vi "Get Attributes.vi"(0 "Linked List in":refnum<class "Linked List.lvclass">, 1 "Unique ID":string, 2 "Include Private?":bool, 3 "Flatten Pointer?":bool, 5 "Attribute Names":string[](array[string]), 7 "Missing GUIDs":string[](array[string]), 9 "Type":variant, 11 "error in (no error)":errorcluster) -> (4 "Linked List out":refnum<class "Linked List.lvclass">, 6 "Attribute Names out":string[](array[string]), 8 "Missing GUIDs out":string[](array[string]), 10 "Attributes":variant[](array[variant]), 12 "Found?":bool[](array[boolean]), 14 "Data IDs":string[](array[string]), 15 "error out":errorcluster)   [LabVIEW 2020, in "Linked Lists.lvlib" / "Linked List.lvclass"]
uses:
  <vilib>/gpm_packages/@cs/linked-list/Source/Linked List/Linked List/Linked List.lvclass
  <vilib>/gpm_packages/@cs/linked-list/Source/Linked List/Linked List Definition/Linked List Definition.lvclass
  <vilib>/gpm_packages/@cs/linked-list/Source/Linked List/Linked List/Linked List.lvclass/Linked List.ctl
  <vilib>/gpm_packages/@cs/lookup-table/Source/LookupTable/LookupTable.lvclass/LookupTable.ctl
  beab1386-fb03-4602-991d-c6dd99164584.vi
  218746c0-9e6e-4e5e-8a67-a9a5cc4de36c.vi
  531c8529-7f46-40ba-a14e-907a47e2dd20.vi
  <vilib>/gpm_packages/@cs/lookup-table/Source/LookupTable/Read Table Reference.vi
  beab1386-fb03-4602-991d-c6dd99164584.vi/5a7267ad-595e-4610-9ac2-8bef780848ff.vi
  218746c0-9e6e-4e5e-8a67-a9a5cc4de36c.vi/5a7267ad-595e-4610-9ac2-8bef780848ff.vi
  531c8529-7f46-40ba-a14e-907a47e2dd20.vi/5a7267ad-595e-4610-9ac2-8bef780848ff.vi
  <vilib>/gpm_packages/@cs/lookup-table/Source/LookupTable/LookupTable.lvclass
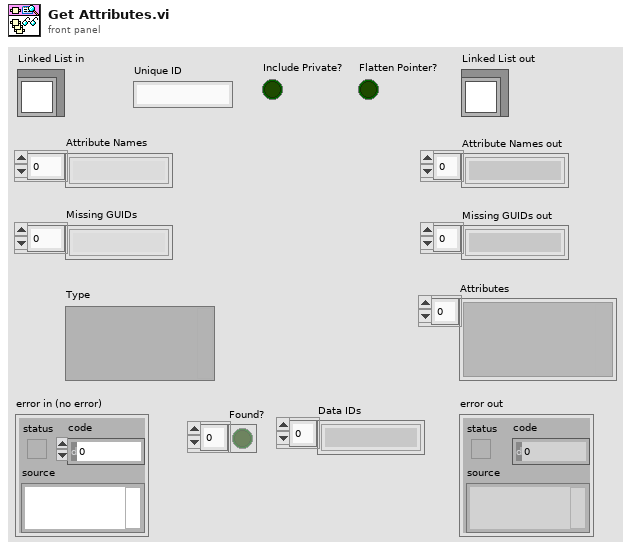
[diagram p1: front panel]
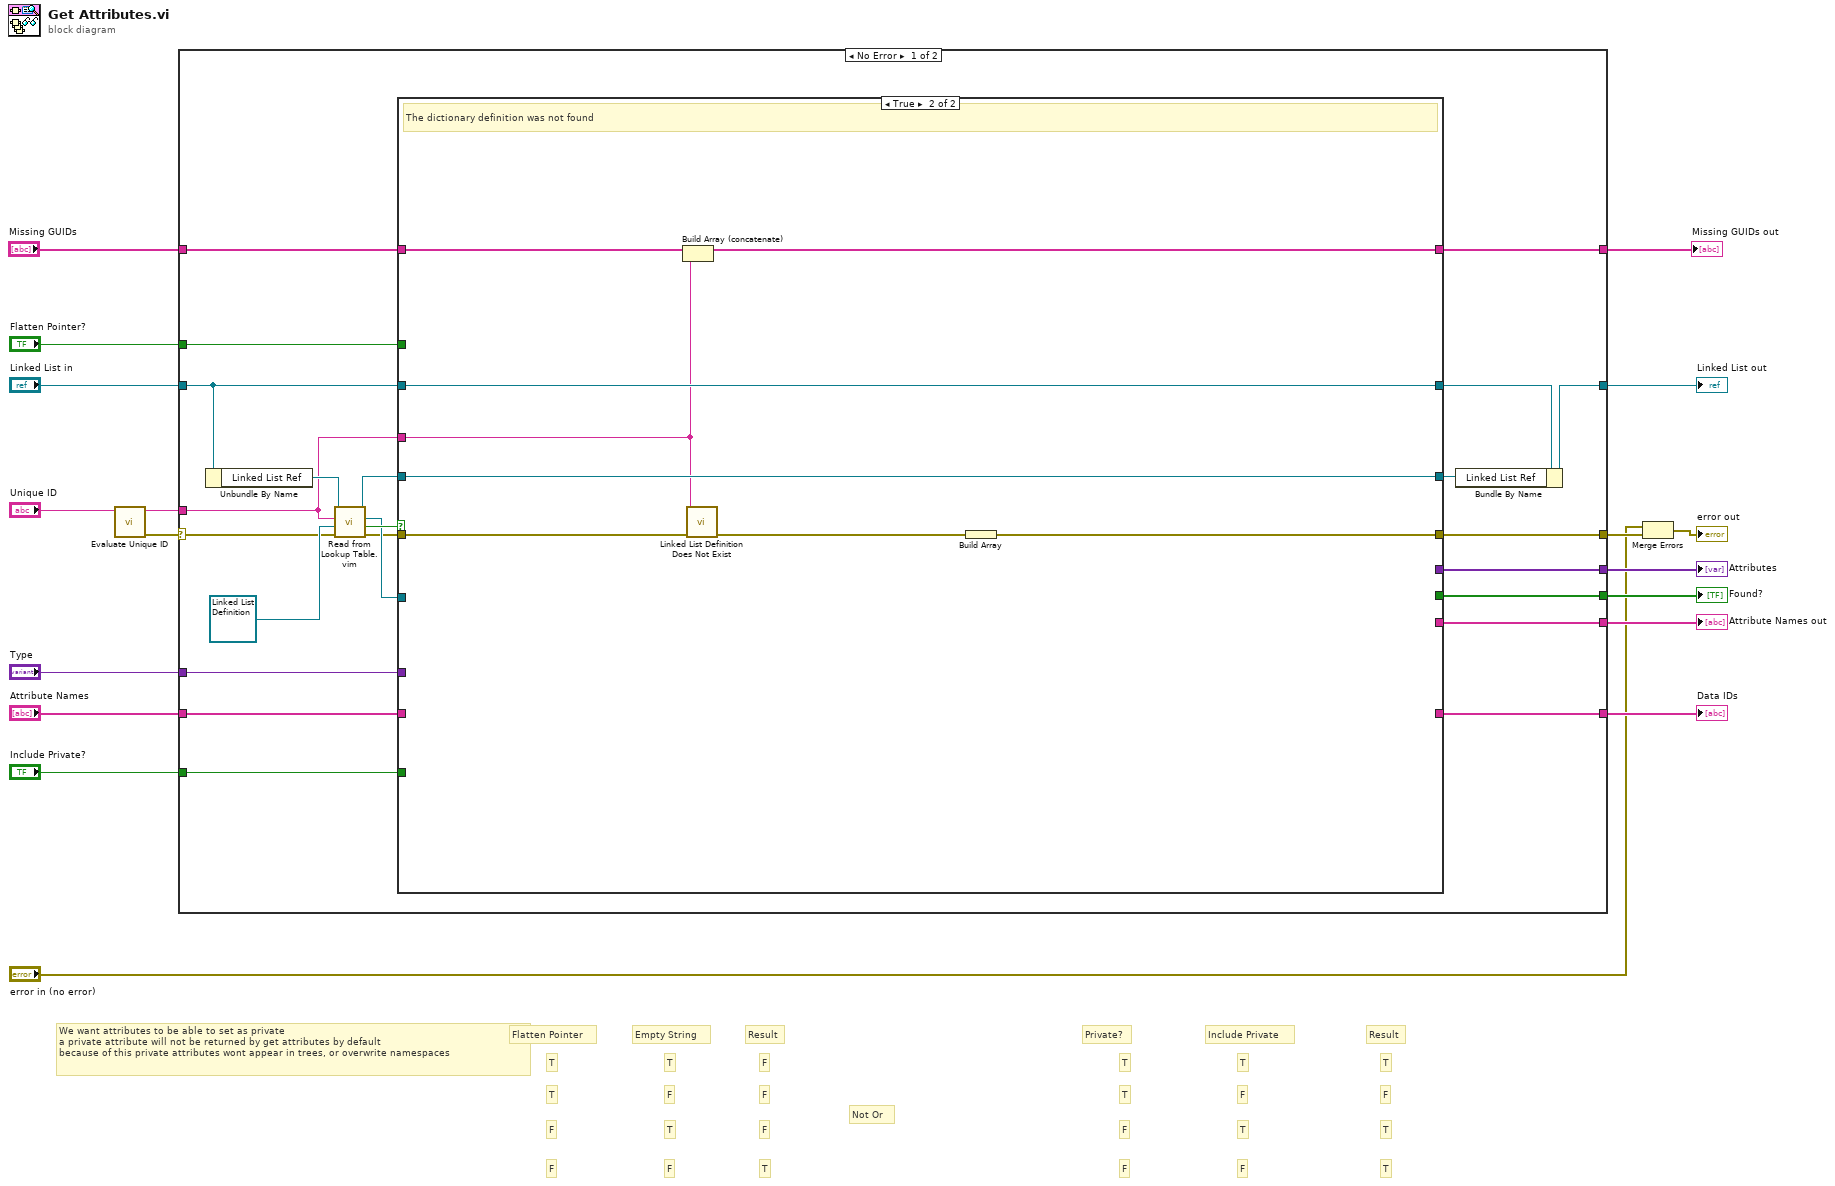
[diagram p0: block diagram]
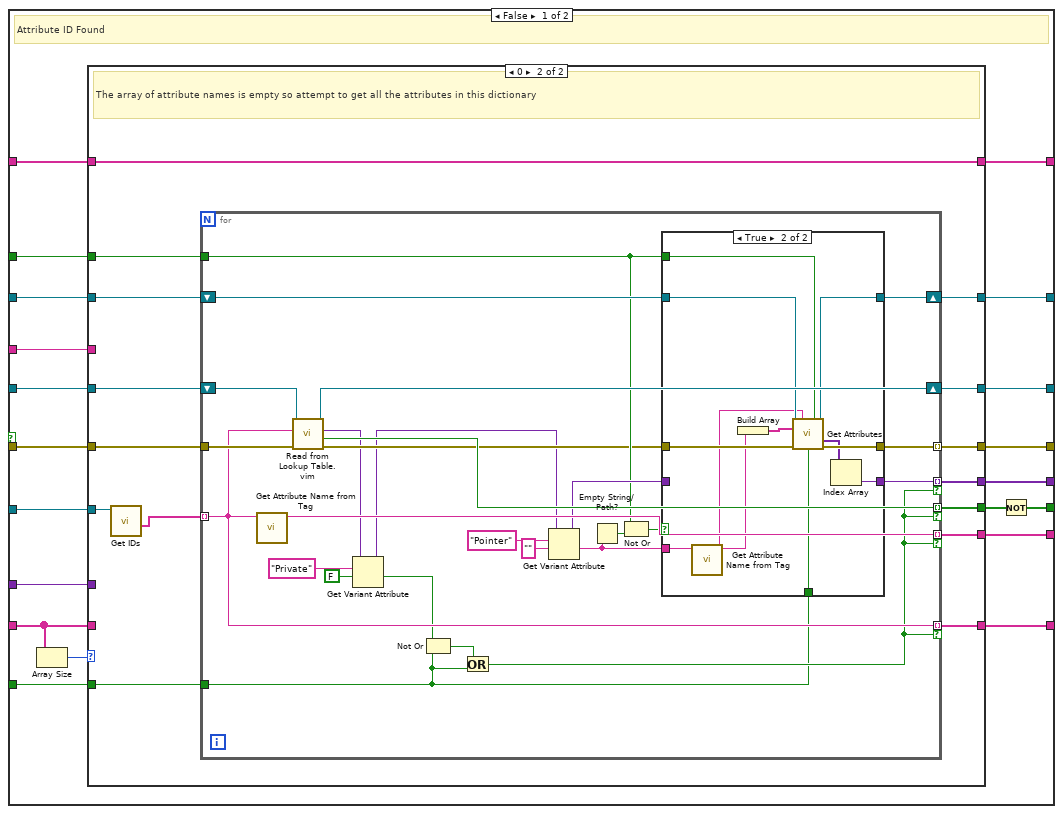
[diagram p2: hidden frame]
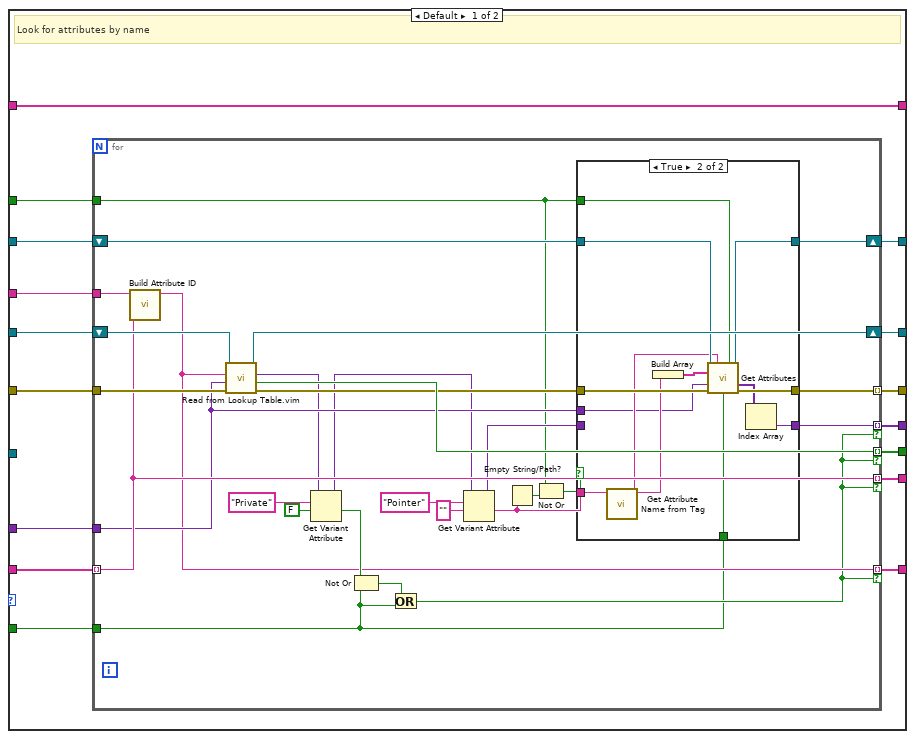
[diagram p3: hidden frame]
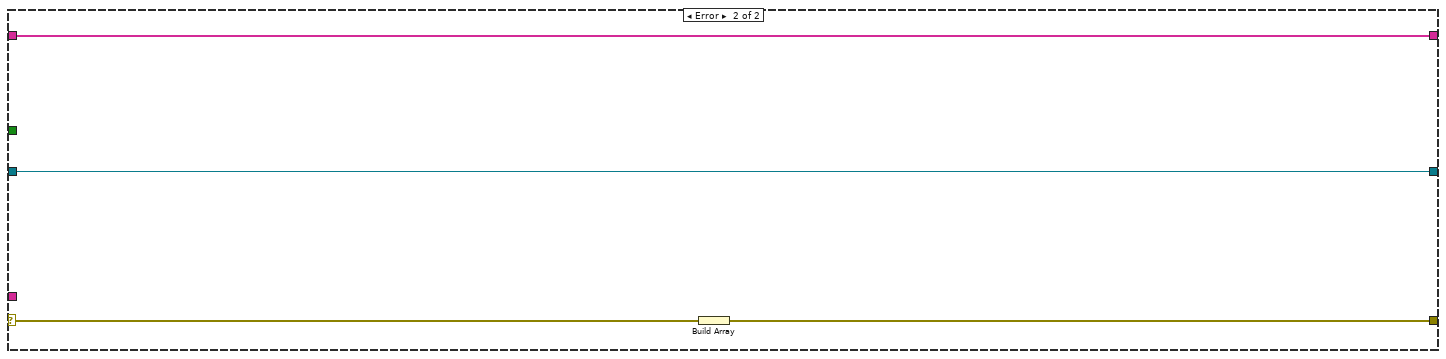
[diagram p6: hidden frame]
diagram:
  # "T"
  # "T"
  # "F"
  # "T"
  # "F"
  # "F"
  # "T"
  # "F"
  # "F"
  # "T"
  # "T"
  # "T"
  # "Result"
  # "Include Private"
  # "Private?"
  # "We want attributes to be able to set as private\na private attribute will not be returned by get attributes by default\nbecause of this private attributes wont appear in trees, or overwrite namespaces"
  # "Not Or"
  # "T"
  # "F"
  # "F"
  # "F"
  # "F"
  # "F"
  # "T"
  # "F"
  # "F"
  # "T"
  # "T"
  # "T"
  # "Result"
  # "Empty String"
  # "Flatten Pointer"
  n1 = call <vilib>:"Evaluate Unique ID.vi"("Unique ID"="Unique ID") -> ("error out"=w15:errorcluster, "Unique ID Out"=w14:string)  [unwired: 9 in]
  n2 = case shown="No Error" w15 {
    selector: w15 -> [w33 w188]
    tunnel: [w34 w189] -> w16
    tunnel: "Linked List in" -> [w24 w189]
    tunnel: w14 -> [w32 _]
    tunnel: [w31 w187] -> w13
    tunnel: "Attribute Names" -> [w30 _]
    tunnel: [w29 _] -> w8
    tunnel: [w28 _] -> w11
    tunnel: [w27 _] -> w10
    tunnel: [w26 _] -> w9
    tunnel: "Type" -> [w25 _]
    tunnel: "Flatten Pointer?" -> [w22 _]
    tunnel: "Include Private?" -> [w21 _]
    tunnel: [w20 w186] -> w2
    tunnel: "Missing GUIDs" -> [w19 w186]
    frame No Error {
      n3 = Unbundle By Name(w24) -> ("Linked List Ref"=w41:refnum<data-value>)
      n4 = call "Read from Lookup Table.vim"("error in (no error)"=w33, "Type"=refnum<class "Linked List Definition.lvclass"> refnum ("Linked List.lvlib:Linked List Definition.lvclass"), "Item Name"=w32, "LookupTable Reference"=w41) -> ("error out"=w36:errorcluster, "Not Found?"=w39:bool, "Value"=w37:refnum<class "Linked List Definition.lvclass">, "LookupTable Reference Out"=w38:refnum<data-value>)  [unwired: 4 in]
      n5 = case shown="True" w39 {
        tunnel: w38 -> [w60 w183]
        tunnel: w37 -> [w58 _]
        tunnel: [w57 w181] -> w31
        tunnel: w36 -> [w61 w185]
        tunnel: w32 -> [w59 w178]
        tunnel: [w56 w183] -> w35
        tunnel: w30 -> [w55 _]
        tunnel: [w53 _] -> w29
        tunnel: [w52 _] -> w28
        tunnel: [w48 _] -> w27
        tunnel: [w50 _] -> w26
        tunnel: w25 -> [w49 _]
        tunnel: [w47 w182] -> w23
        tunnel: w24 -> [w46 w182]
        tunnel: w22 -> [w45 _]
        tunnel: w21 -> [w44 _]
        tunnel: [w43 w179] -> w20
        tunnel: w19 -> [w42 w180]
        frame False {
          # "Attribute ID Found"
          n6 = Array Size(array=w55) -> (size(s)=w54:i32)
          n7 = case shown="0" w54 {
            tunnel: w61 -> [w75 w136]
            tunnel: w60 -> [w77 w135]
            tunnel: w59 -> [w72 _]
            tunnel: w58 -> [_ w132]
            tunnel: [w74 w134] -> w57
            tunnel: [w76 w133] -> w56
            tunnel: w55 -> [w73 _]
            tunnel: [w71 w125] -> w53
            tunnel: [w68 w131] -> w52
            tunnel: [w69 w128] -> w51
            tunnel: [w70 w130] -> w50
            tunnel: w49 -> [w67 _]
            tunnel: [w65 w126] -> w47
            tunnel: w46 -> [w66 w127]
            tunnel: w45 -> [w64 w124]
            tunnel: w44 -> [w63 w123]
            tunnel: [w62 w122] -> w43
            tunnel: w42 -> [w62 w122]
            frame Default {
              # "Look for attributes by name"
              n8 = for {
                shift-right: [w102] -> w76
                shift-left: w77 -> [w103]
                tunnel: w73 -> [w100] mode=indexing
                tunnel: w72 -> [w105]
                tunnel: [w80] -> w71 mode=indexing if=w79
                tunnel: [w100] -> w70 mode=indexing if=w79
                tunnel: [w101] -> w69 mode=indexing if=w79
                tunnel: [w90] -> w68 mode=indexing if=w79
                tunnel: w67 -> [w92]
                shift-right: [w94] -> w65
                shift-left: w66 -> [w95]
                tunnel: w64 -> [w88]
                tunnel: w63 -> [w78]
                tunnel: w75 -> [w104]
                tunnel: [w96] -> w74 mode=indexing
                n9 = call <vilib>:"Build Attribute ID.vi"("Attr Name"=w100, "Unique ID"=w105) -> ("Attr ID Out"=w80:string)  [unwired: 9 in]
                n10 = call "Read from Lookup Table.vim"("error in (no error)"=w104, "Type"=w92, "Item Name"=w80, "LookupTable Reference"=w103) -> ("error out"=w97:errorcluster, "Not Found?"=w101:bool, "Value"=w86:variant, "LookupTable Reference Out"=w102:refnum<data-value>)  [unwired: 4 in]
                n11 = Get Variant Attribute(Variant=w86, name="Private", default value (empty Variant)=FALSE) -> (duplicate Variant=w85:variant, value=w82:bool)  [unwired: 1 in, 2 out]
                n12 = Not Or(1:w78, 2:w82) -> (0:w81:bool)
                n13 = Or(x=w81, y=w78) -> (x .or. y?=w79:bool)
                n14 = Get Variant Attribute(Variant=w85, name="Pointer", default value (empty Variant)="") -> (duplicate Variant=w91:variant, value=w93:string)  [unwired: 1 in, 2 out]
                n15 = Empty String/Path?(string/path=w93) -> (empty?=w89:bool)
                n16 = Not Or(1:w89, 2:w88) -> (0:w87:bool)
                n17 = case shown="True" w87 {
                  tunnel: w97 -> [w107 w121]
                  tunnel: [w107 w120] -> w96
                  tunnel: w95 -> [w108 w119]
                  tunnel: [w108 w118] -> w94
                  tunnel: w88 -> [_ w117]
                  tunnel: w93 -> [_ w116]
                  tunnel: w92 -> [_ w112]
                  tunnel: [w106 w110] -> w90
                  tunnel: w91 -> [w106 _]
                  tunnel: w78 -> [_ w109]
                  frame False {
                  }
                  frame True {
                    n18 = call <vilib>:"Get Attribute Name from Tag.vi"("Tag"=w116) -> ("Linked List ID"=w115:string, "Attribute Name"=w114:string)  [unwired: 8 in, 1 out]
                    n19 = Build Array(w114) -> (w113:string[])
                    n20 = call <vilib>:"Get Attributes.vi"("Linked List in"=w119, "Unique ID"=w115, "Include Private?"=w109, "Flatten Pointer?"=w117, "Attribute Names"=w113, "Type"=w112, "error in (no error)"=w121) -> ("Linked List out"=w118:refnum<class "Linked List.lvclass">, "Attributes"=w111:variant[], "error out"=w120:errorcluster)  [unwired: 2 in, 4 out]
                    n21 = Index Array(array=w111) -> (element=w110:variant)  [unwired: 1 in]
                  }
                }
              }
            }
            frame 0 {
              # "The array of attribute names is empty so attempt to get all the attributes in this dictionary"
              n22 = call <vilib>:"Get IDs.vi"("Linked List Definition in"=w132) -> ("Data IDs"=w129:string[])  [unwired: 8 in, 2 out]
              n23 = for {
                shift-right: [w160] -> w133
                shift-left: w135 -> [w161]
                tunnel: w129 -> [w157] mode=indexing
                tunnel: [w146] -> w131 mode=indexing if=w138
                tunnel: [w159] -> w128 mode=indexing if=w138
                tunnel: [w158] -> w130 mode=indexing if=w138
                shift-right: [w149] -> w126
                shift-left: w127 -> [w150]
                tunnel: [w157] -> w125 mode=indexing if=w138
                tunnel: w124 -> [w148]
                tunnel: w123 -> [w137]
                tunnel: w136 -> [w162]
                tunnel: [w145] -> w134 mode=indexing
                n24 = call <vilib>:"Get Attribute Name from Tag.vi"("Tag"=w157) -> ("Attribute Name"=w158:string)  [unwired: 8 in, 2 out]
                n25 = call "Read from Lookup Table.vim"("error in (no error)"=w162, "Item Name"=w157, "LookupTable Reference"=w161) -> ("error out"=w147:errorcluster, "Not Found?"=w159:bool, "Value"=w140:variant, "LookupTable Reference Out"=w160:refnum<data-value>)  [unwired: 5 in]
                n26 = Get Variant Attribute(Variant=w140, name="Private", default value (empty Variant)=FALSE) -> (duplicate Variant=w139:variant, value=w142:bool)  [unwired: 1 in, 2 out]
                n27 = Not Or(1:w137, 2:w142) -> (0:w141:bool)
                n28 = Or(x=w141, y=w137) -> (x .or. y?=w138:bool)
                n29 = Get Variant Attribute(Variant=w139, name="Pointer", default value (empty Variant)="") -> (duplicate Variant=w153:variant, value=w154:string)  [unwired: 1 in, 2 out]
                n30 = Empty String/Path?(string/path=w154) -> (empty?=w152:bool)
                n31 = Not Or(1:w152, 2:w148) -> (0:w151:bool)
                n32 = case shown="True" w151 {
                  tunnel: w147 -> [w164 w177]
                  tunnel: [w164 w176] -> w145
                  tunnel: w150 -> [w165 w175]
                  tunnel: [w165 w174] -> w149
                  tunnel: w148 -> [_ w173]
                  tunnel: w154 -> [_ w172]
                  tunnel: [w163 w167] -> w146
                  tunnel: w153 -> [w163 _]
                  tunnel: w137 -> [_ w166]
                  frame False {
                  }
                  frame True {
                    n33 = call <vilib>:"Get Attribute Name from Tag.vi"("Tag"=w172) -> ("Linked List ID"=w171:string, "Attribute Name"=w170:string)  [unwired: 8 in, 1 out]
                    n34 = Build Array(w170) -> (w169:string[])
                    n35 = call <vilib>:"Get Attributes.vi"("Linked List in"=w175, "Unique ID"=w171, "Include Private?"=w166, "Flatten Pointer?"=w173, "Attribute Names"=w169, "error in (no error)"=w177) -> ("Linked List out"=w174:refnum<class "Linked List.lvclass">, "Attributes"=w168:variant[], "error out"=w176:errorcluster)  [unwired: 3 in, 4 out]
                    n36 = Index Array(array=w168) -> (element=w167:variant)  [unwired: 1 in]
                  }
                }
              }
            }
          }
          n37 = Not(x=w51) -> (.not. x?=w48:bool[])
        }
        frame True {
          # "The dictionary definition was not found"
          n38 = Build Array (concatenate)(w180, w178) -> (w179:string[])
          n39 = call <vilib>:"Linked List Definition Does Not Exist.vi"("Error In"=w185, "Unique ID"=w178) -> ("Error Out"=w184:errorcluster)  [unwired: 9 in]
          n40 = Build Array(w184) -> (w181:errorcluster[])
        }
      }
      n41 = Bundle By Name(cluster=w23, "Linked List Ref"=w35) -> (w34:refnum<class "Linked List.lvclass">)
    }
    frame Error {
      n42 = Build Array(w188) -> (w187:errorcluster[])
    }
  }
  "Linked List out" <- w16
  "Attributes" <- w11
  "Found?" <- w10
  "Attribute Names out" <- w9
  "Data IDs" <- w8
  "Missing GUIDs out" <- w2
  n43 = Merge Errors("error in (no error)", w13) -> (→"error out":errorcluster)
